vi "GetLocnsAndSave.vi"   [LabVIEW 2020]
panel:
  # "Save FP Locations"
  # "Gets the locations of of all currently loaded Front Panels and saves them to a file of your choosing, stored by default  in the \"LabVIEW Data folder\""
types:
  T1 = typedef "VInameSizePath.ctl" = cluster{"VI Name":string, "Front Panel.WinBounds":T2, "File Path":path}
  T2 = typedef "LVRectTypeDef.ctl" = cluster{"Left":i16, "Top":i16, "Right":i16, "Bottom":i16}
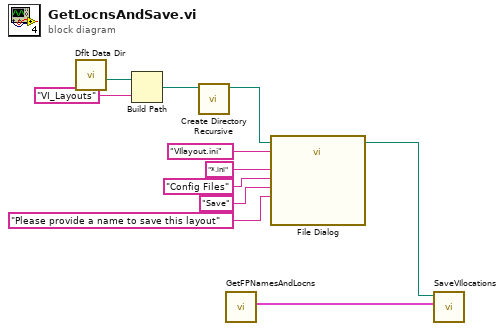
[diagram p0: block diagram]
diagram:
  n1 = call <vilib>:"Dflt Data Dir.vi"() -> ("App:Default Data Directory"=w9:path)
  n2 = Build Path(base path=w9, name or relative path="VI_Layouts") -> (appended path=w2:path)
  n3 = call <vilib>:"Create Directory Recursive.vi"("directory"=w2) -> ("directory copy"=w1:path)  [unwired: 4 in, 2 out]
  n4 = call "GetFPNamesAndLocns.vi"() -> ("Array"=w11:T1[])  [unwired: 11 in]
  n5 = call "File Dialog"("start path"=w1, "prompt"="Please provide a name to save this layout", "button label"="Save", "default name"="VIlayout.ini", "pattern (all files)"="*.ini", "pattern label"="Config Files" ("button label")) -> ("selected path"=w10:path)  [unwired: 6 in, 3 out]
  n6 = call "SaveVIlocations.vi"("NamesAndLocnsArray"=w11, "configuration file path"=w10) -> ()  [unwired: 10 in]
